vi "ley_de_senos.vi"(9 "ady2":dbl, 10 "opuesto":dbl, 11 "ady1":dbl) -> (3 "angulo":dbl)   [LabVIEW 2017]
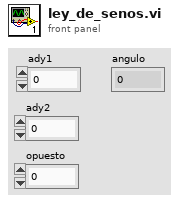
[diagram p1: front panel]
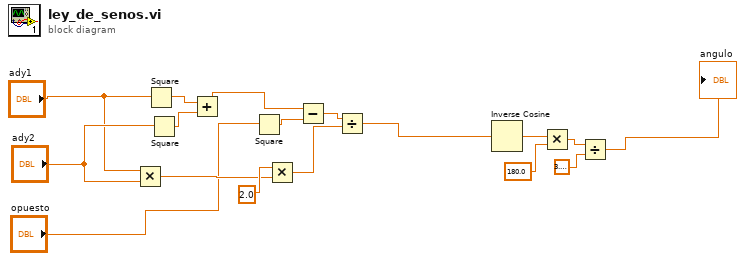
[diagram p0: block diagram]
diagram:
  n1 = Multiply(x="ady1", y="ady2") -> (x*y=w7:dbl)
  n2 = Square(x="ady1") -> (x^2=w2:dbl)
  n3 = Square(x="ady2") -> (x^2=w3:dbl)
  n4 = Add(x=w2, y=w3) -> (x+y=w11:dbl)
  n5 = Square(x="opuesto") -> (x^2=w10:dbl)
  n6 = Multiply(x=2.0, y=w7) -> (x*y=w9:dbl)
  n7 = Subtract(x=w11, y=w10) -> (x-y=w4:dbl)
  n8 = Divide(x=w4, y=w9) -> (x/y=w12:dbl)
  n9 = Inverse Cosine(1:w12) -> (0:w13:dbl)
  n10 = Multiply(x=w13, y=180.0) -> (x*y=w15:dbl)
  n11 = Divide(x=w15, y=3.141592653589793) -> (x/y=→"angulo":dbl)
